vi "ICNC Write EEPROM.vi"(6 "TimeOut":u32, 7 "WaitCompletion":i32, 8 "error in (no error)":errorcluster caption="entrée d'erreur (pas d'erreur)", 9 "Value":string, 10 "Length":u32, 11 "StartAdress":u32) -> (0 "error out":errorcluster caption="sortie d'erreur", 1 "Value out":string, 3 "function return":u32)   [LabVIEW 2012, in "ICNC2.lvlib"]
doc: "DWORD ICNC_WriteEEPROM( DWORD StartAdress,\n DWORD Length,\n BYTE* Value,\n BOOL WaitCompletion=TRUE,\n DWORD TimeOut=1000);"
uses:
  <userlib>/ICNC/ICNC2.lvlib
  <userlib>/ICNC/ICNC2.dll
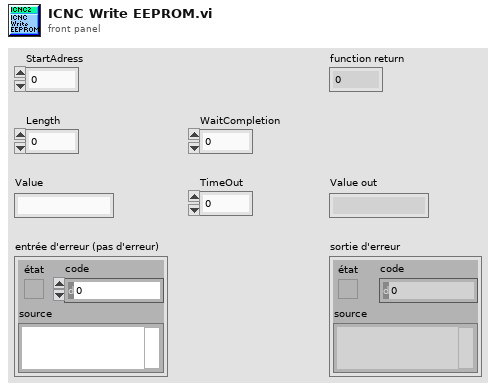
[diagram p1: front panel]
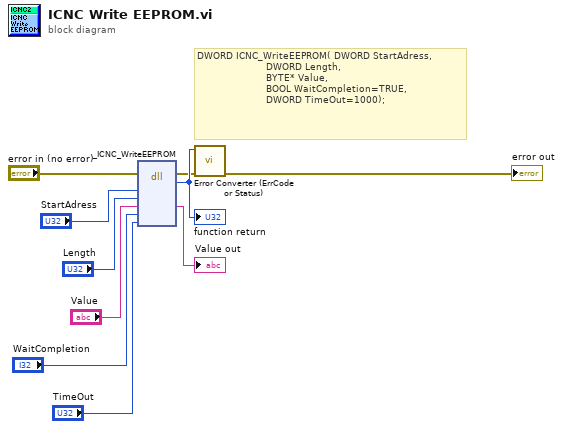
[diagram p0: block diagram]
diagram:
  # "DWORD ICNC_WriteEEPROM( DWORD StartAdress,\n                       DWORD Length,\n                       BYTE* Value,\n                       BOOL WaitCompletion=TRUE,\n                       DWORD TimeOut=1000);"
  n1 = dll-call lib="C:/Program Files (x86)/National Instruments/LabVIEW 2012/user.lib/ICNC/ICNC2.*" fn="_ICNC_WriteEEPROM"(error in="error in (no error)", "StartAdress"="StartAdress", "Length"="Length", "Value"="Value", "WaitCompletion"="WaitCompletion", "TimeOut"="TimeOut") -> (error out=w2:errorcluster, w10:u32, "Value"=→"Value out":string)  [unwired: 6 in, 1 out]
  "function return" <- w10
  n2 = call <userlib>:"Error Converter (ErrCode or Status).vi"("error in (no error)"=w2, "error code"=w10) -> ("error out"=→"error out":errorcluster)  [unwired: 9 in]
